vi "RGImageOverlay.vi"(7 "RGB_Image":T2, 8 "Error In":errorcluster, 9 "Overlay?":bool, 10 "UI Controls Refnum":T3, 11 "Image Input Cluster":T1) -> (0 "Error Out":errorcluster, 3 "Saved Image":T2)   [LabVIEW 2012]
doc: "SciScan 1.2 160622"
uses:
  <vilib>/vision/Image Controls.llb/IMAQ Image.ctl
  Custom Control and Typedefs/UI Controls Refnum.ctl
  Custom Control and Typedefs/ChannelSelector_for_PosSave.ctl
  Custom Controls/PositionSaveMod.ctl
  Custom Control and Typedefs/Overlay Control.ctl
  Custom Control and Typedefs/ImageCluster.ctl
  <vilib>/vision/NI_Vision_Development_Module.lvlib
panel:
  out "error out":errorcluster
  # "Red (Current Image)"
  # "Green (Saved Image)"
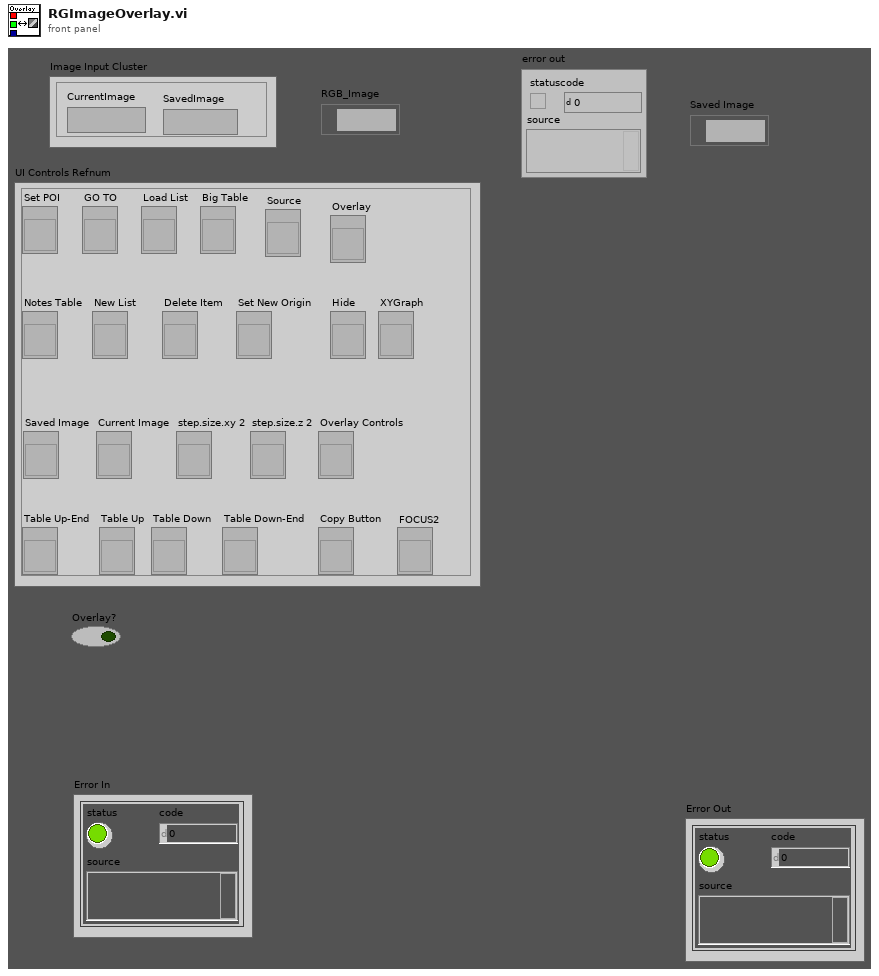
[diagram p1: front panel]
types:
  T1 = typedef "ImageCluster.ctl" = cluster{"CurrentImage":T2, "SavedImage":T2}
  T2 = typedef "IMAQ Image.ctl" = refnum<image>
  T3 = typedef "UI Controls Refnum.ctl" = cluster{"GO TO":refnum<vi>, "Load List":refnum<vi>, "Big Table":refnum<vi>, "Notes Table":refnum<vi>, "New List":refnum<vi>, "Delete Item":refnum<vi>, "Set New Origin":refnum<vi>, "Set POI":refnum<vi>, "Saved Image":refnum<vi>, "Current Image":refnum<vi>, "step.size.xy 2":refnum<vi>, "step.size.z 2":refnum<vi>, "Source":refnum<vi>, "Table Up-End":refnum<vi>, "Table Up":refnum<vi>, "Table Down":refnum<vi>, "Table Down-End":refnum<vi>, "Copy Button":refnum<vi>, "Hide":refnum<vi>, "Overlay Controls":refnum<vi>, "Overlay":refnum<vi>, "XYGraph":refnum<vi>, "FOCUS2":refnum<vi>}
  T4 = typedef "Overlay Control.ctl" = cluster{"auto scale\n      Red ":bool, "Min Max Saved (Green)":cluster{dbl, dbl}, "auto scale\n      Green":bool, "Min Max Saved (Red)":cluster{dbl, dbl}}
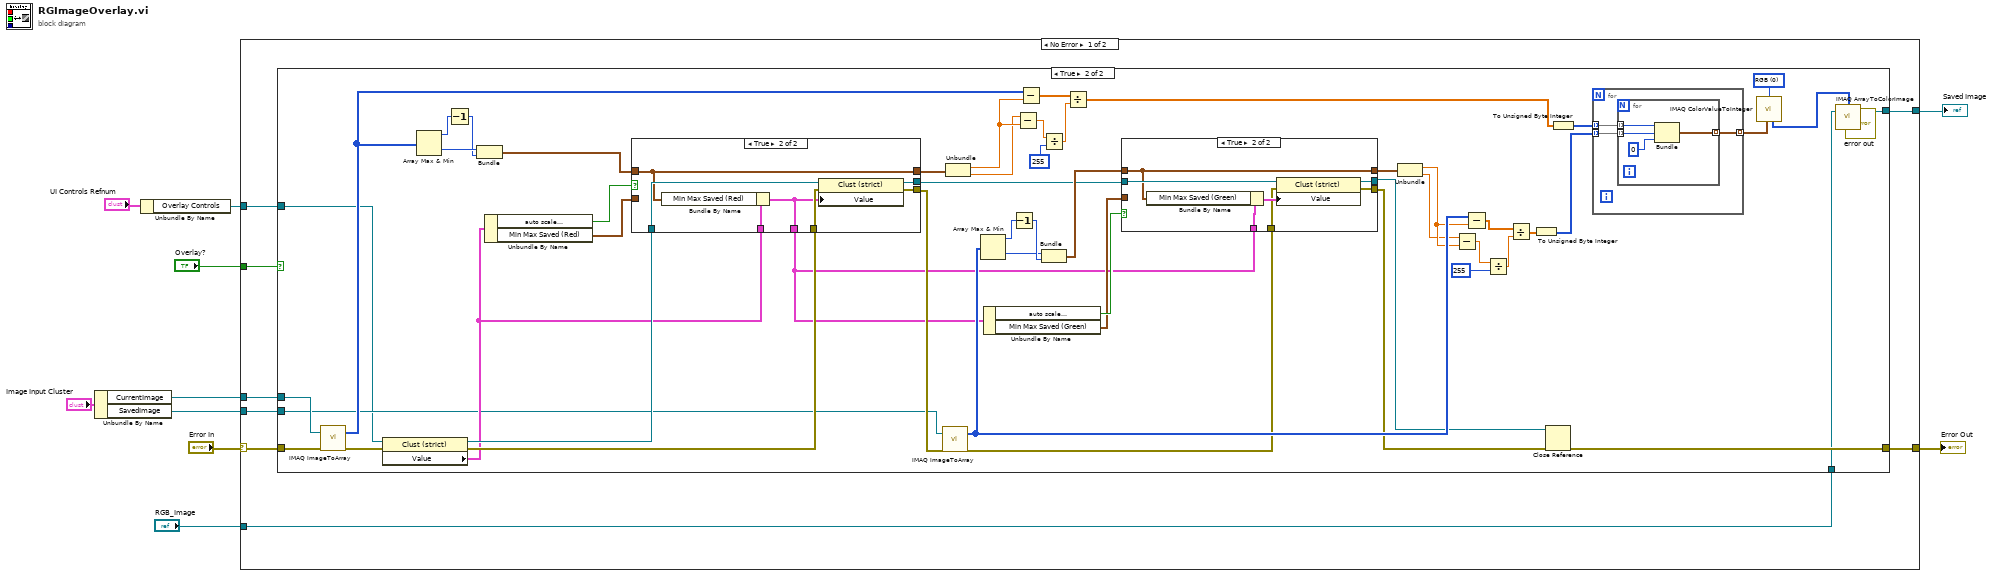
[diagram p0: block diagram]
diagram:
  n1 = Unbundle By Name("Image Input Cluster") -> ("CurrentImage"=w8:T2, "SavedImage"=w7:T2)
  n2 = Unbundle By Name("UI Controls Refnum") -> ("Overlay Controls"=w5:refnum<vi>)
  n3 = case shown="No Error" "Error In" {
    selector: "Error In" -> [w17 w102]
    tunnel: [w14 w102] -> w10
    tunnel: w8 -> [w18 _]
    tunnel: w7 -> [w16 w103]
    tunnel: [w15 w103] -> w6
    tunnel: w5 -> [w13 _]
    tunnel: "Overlay?" -> [w12 _]
    tunnel: "RGB_Image" -> [w11 _]
    frame No Error {
      n4 = case shown="True" w12 {
        tunnel: w18 -> [_ w58]
        tunnel: w17 -> [w19 w57]
        tunnel: w16 -> [w20 w29]
        tunnel: [w20 w28] -> w15
        tunnel: [w19 w25] -> w14
        tunnel: w13 -> [_ w24]
        tunnel: w11 -> [_ w23]
        frame False {
        }
        frame True {
          w60 = u16 0 items=["RGB", "HSL", "HSV", "HSI"] ("Color Mode")
          n5 = call "IMAQ ImageToArray"("error in (no error)"=w57, "Image"=w58) -> ("error out"=w52:errorcluster, "Image Pixels (I16)"=w53:i16[][])  [unwired: 2 in, 3 out]
          n6 = property class="Clust (strict)"(reference=w24, error in=w52) -> (reference out=w48:refnum<vi>, error out=w44:errorcluster, "Value"=w34:T4)
          n7 = Array Max & Min(array=w53) -> (max value=w56:i16, min value=w55:i16)  [unwired: 2 out]
          n8 = Decrement(x=w56) -> (x-1=w54:i16)
          n9 = Bundle(w55, w54) -> (w50:cluster{i16, i16})  [unwired: 1 in]
          n10 = Unbundle By Name(w34) -> ("auto scale\n      Red"=w51:bool, "Min Max Saved (Red)"=w49:cluster{dbl, dbl})
          n11 = case shown="True" w51 {
            tunnel: w50 -> [_ w92]
            tunnel: w49 -> [w87 _]
            tunnel: w48 -> [w85 w94]
            tunnel: w34 -> [w84 w93]
            tunnel: [w87 w92] -> w47
            tunnel: [w85 w91] -> w36
            tunnel: w44 -> [w86 w90]
            tunnel: [w86 w89] -> w43
            tunnel: [w84 w88] -> w22
            frame False {
            }
            frame True {
              n12 = Bundle By Name(cluster=w93, "Min Max Saved (Red)"=w92) -> (w88:T4)
              n13 = property class="Clust (strict)"(reference=w94, error in=w90, "Value"=w88) -> (reference out=w91:refnum<vi>, error out=w89:errorcluster)
            }
          }
          n14 = call "IMAQ ImageToArray"("error in (no error)"=w43, "Image"=w29) -> ("error out"=w33:errorcluster, "Image Pixels (I16)"=w39:i16[][])  [unwired: 2 in, 3 out]
          n15 = Unbundle(w47) -> (w46:dbl, w45:dbl)
          n16 = Array Max & Min(array=w39) -> (max value=w40:i16, min value=w41:i16)  [unwired: 2 out]
          n17 = Unbundle By Name(w22) -> ("auto scale\n      Green"=w37:bool, "Min Max Saved (Green)"=w35:cluster{dbl, dbl})
          n18 = Decrement(x=w40) -> (x-1=w42:i16)
          n19 = Subtract(x=w45, y=w46) -> (x-y=w64:dbl)
          n20 = Subtract(x=w53, y=w46) -> (x-y=w73:dbl[][])
          n21 = Bundle(w41, w42) -> (w38:cluster{i16, i16})  [unwired: 1 in]
          n22 = Divide(x=w64, y=i16 255) -> (x/y=w72:dbl)
          n23 = Divide(x=w73, y=w72) -> (x/y=w70:dbl[][])
          n24 = case shown="True" w37 {
            tunnel: w38 -> [_ w80]
            tunnel: w35 -> [w76 _]
            tunnel: w36 -> [w74 w83]
            tunnel: w22 -> [_ w82]
            tunnel: [w76 w80] -> w32
            tunnel: [w74 w79] -> w26
            tunnel: w33 -> [w75 w78]
            tunnel: [w75 w77] -> w27
            frame False {
            }
            frame True {
              n25 = Bundle By Name(cluster=w82, "Min Max Saved (Green)"=w80) -> (w81:T4)
              n26 = property class="Clust (strict)"(reference=w83, error in=w78, "Value"=w81) -> (reference out=w79:refnum<vi>, error out=w77:errorcluster)
            }
          }
          n27 = Unbundle(w32) -> (w31:dbl, w30:dbl)
          n28 = Subtract(x=w30, y=w31) -> (x-y=w65:dbl)
          n29 = Subtract(x=w39, y=w31) -> (x-y=w66:dbl[][])
          n30 = Divide(x=w65, y=i16 255) -> (x/y=w67:dbl)
          n31 = Divide(x=w66, y=w67) -> (x/y=w69:dbl[][])
          n32 = To Unsigned Byte Integer(number=w69) -> (unsigned 8bit integer=w62:u8[][])
          n33 = Close Reference(reference=w26, error in (no error)=w27) -> (error out=w25:errorcluster)
          n34 = To Unsigned Byte Integer(number=w70) -> (unsigned 8bit integer=w63:u8[][])
          n35 = for {
            tunnel: w63 -> [w96] mode=indexing
            tunnel: w62 -> [w97] mode=indexing
            tunnel: [w95] -> w61 mode=indexing
            n36 = for {
              tunnel: w97 -> [w98] mode=indexing
              tunnel: w96 -> [w101] mode=indexing
              tunnel: [w100] -> w95 mode=indexing
              n37 = Bundle(w101, w98, u8 0) -> (w100:cluster{u8, u8, u8})  [unwired: 1 in]
            }
          }
          n38 = call "IMAQ ColorValueToInteger"("2D Color value array"=w61, "Color Mode"=w60) -> ("2D U32 array"=w59:u32[][])  [unwired: 3 in, 3 out]
          n39 = call "IMAQ ArrayToColorImage"("Image Pixels (U32)"=w59, "Image"=w23) -> ("Image Out"=w28:T2, "error out"=→"error out":errorcluster)  [unwired: 3 in]
        }
      }
    }
    frame Error {
    }
  }
  "Error Out" <- w10
  "Saved Image" <- w6
